vi "SetIDSN(SubVI).vi"(8 "input sn":string, 11 "sn":string) -> (2 "output frame":string)   [LabVIEW 2012]
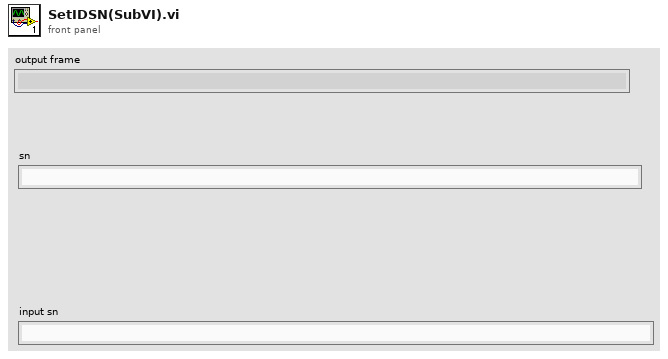
[diagram p1: front panel]
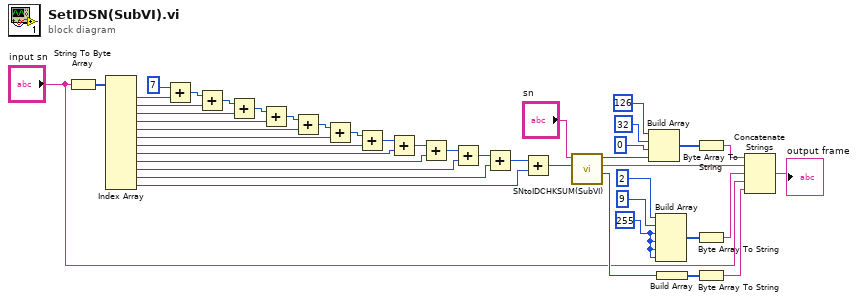
[diagram p0: block diagram]
diagram:
  w33 = u8 255
  n1 = String To Byte Array(string="input sn") -> (unsigned byte array=w28:u8[])
  n2 = Index Array(array=w28) -> (element #1=w27:u8, element #2=w26:u8, element #3=w25:u8, element #4=w24:u8, element #5=w23:u8, element #6=w22:u8, element #7=w21:u8, element #8=w20:u8, element #9=w19:u8, element #10=w18:u8, element #11=w17:u8, element #12=w16:u8)  [unwired: 12 in]
  n3 = Add(x=u8 7, y=w27) -> (x+y=w5:u8)
  n4 = Add(x=w5, y=w26) -> (x+y=w6:u8)
  n5 = Add(x=w6, y=w25) -> (x+y=w7:u8)
  n6 = Add(x=w7, y=w24) -> (x+y=w8:u8)
  n7 = Add(x=w8, y=w23) -> (x+y=w9:u8)
  n8 = Add(x=w9, y=w22) -> (x+y=w10:u8)
  n9 = Add(x=w10, y=w21) -> (x+y=w11:u8)
  n10 = Add(x=w11, y=w20) -> (x+y=w12:u8)
  n11 = Add(x=w12, y=w19) -> (x+y=w13:u8)
  n12 = Add(x=w13, y=w18) -> (x+y=w14:u8)
  n13 = Add(x=w14, y=w17) -> (x+y=w15:u8)
  n14 = Add(x=w15, y=w16) -> (x+y=w4:u8)
  n15 = call "SNtoIDCHKSUM(SubVI).vi"("fix cheksum"=w4, "input sn"="sn") -> ("output check sum"=w29:u8, "output sn"=w42:string, "output id"=w39:u8)  [unwired: 7 in]
  n16 = Build Array(u8 126, u8 32, u8 0, w39) -> (w40:u8[])
  n17 = Build Array(u8 2, u8 9, w33, w33, w33, w33) -> (w31:u8[])
  n18 = Build Array(w29) -> (w32:u8[])
  n19 = Byte Array To String(unsigned byte array=w40) -> (string=w41:string)
  n20 = Byte Array To String(unsigned byte array=w31) -> (string=w30:string)
  n21 = Byte Array To String(unsigned byte array=w32) -> (string=w1:string)
  n22 = Concatenate Strings(w41, w42, w30, "input sn", w1) -> (→"output frame":string)
